vi "Check_Status_2_tl.vi"(0 "Status Request Reply":string) -> (1 "Status Strings":string, 2 "Error?":bool, 3 "Keep Checking?":bool, 4 "Stopped?":bool, 5 "Current Position":i32)   [LabVIEW 2010]
panel:
  in  "?":cluster{string, "Status Byte":u32}[](array[cluster])=[{"Running program", "Status Byte"=1}, {"Doing Move", "Status Byte"=2}, {"Fwd Lim !", "Status Byte"=4}, {"Rev Lim !", "Status Byte"=8}, {"Home", "Status Byte"=16}, {"Error stopping...!", "Status Byte"=32}, {"Stopped:", "Status Byte"=64}, {"Stopped on Error!", "Status Byte"=128}] {"Status Byte" format="%.0x"}
  out "Status Byte":u32 format="%.0x"
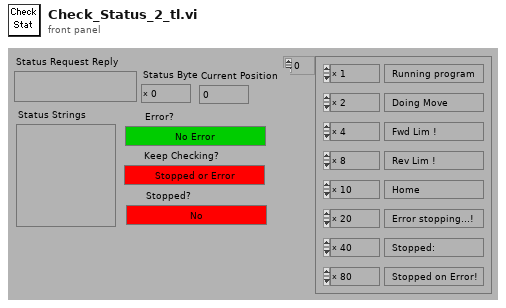
[diagram p1: front panel]
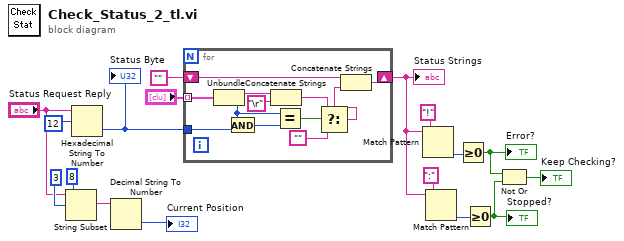
[diagram p0: block diagram]
diagram:
  n1 = String Subset(string="Status Request Reply", offset (0)=3, length (rest)=8) -> (substring=w6:string)
  n2 = Hexadecimal String To Number(string="Status Request Reply", offset=12) -> (number=w15:u32)  [unwired: 1 in, 1 out]
  "Status Byte" <- w15
  n3 = Decimal String To Number(string=w6) -> (number=→"Current Position":i32)  [unwired: 2 in, 1 out]
  n4 = for {
    tunnel: "?" -> [w28] mode=indexing
    tunnel: w15 -> [w26]
    shift-right: [w22] -> w9
    shift-left: "" -> [w23]
    n5 = Unbundle(w28) -> (w20:string, "Status Byte"=w27:u32)
    n6 = And(x=w27, y=w26) -> (x .and. y?=w29:u32)
    n7 = Concatenate Strings(w20, "\r") -> (w18:string)
    n8 = Equal?(x=w27, y=w29) -> (x = y?=w25:bool)
    n9 = Select(t=w18, s=w25, f="") -> (s? t:f=w21:string)
    n10 = Concatenate Strings(w23, w21) -> (w22:string)
  }
  "Status Strings" <- w9
  n11 = Match Pattern(string=w9, regular expression="!") -> (offset past match=w12:i32)  [unwired: 1 in, 3 out]
  n12 = Match Pattern(string=w9, regular expression=":") -> (offset past match=w11:i32)  [unwired: 1 in, 3 out]
  n13 = Greater Or Equal To 0?(x=w12) -> (x >= 0?=w1:bool)
  "Error?" <- w1
  n14 = Greater Or Equal To 0?(x=w11) -> (x >= 0?=w2:bool)
  "Stopped?" <- w2
  n15 = Not Or(1:w2, 2:w1) -> (0:→"Keep Checking?":bool)
